vi "Date Format checkvi.vi"(1 "Date String In":string) -> (0 "Corrected Date":string)   [LabVIEW 2020]
panel:
  out "Day":string
  out "Month":string
  out "Year":string
  out "The separators are correct?":bool
  out "The year is correct?":bool
  out "The length is correct?":bool
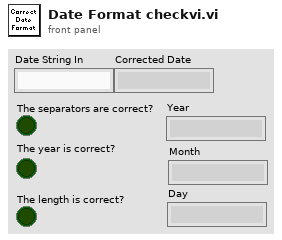
[diagram p1: front panel]
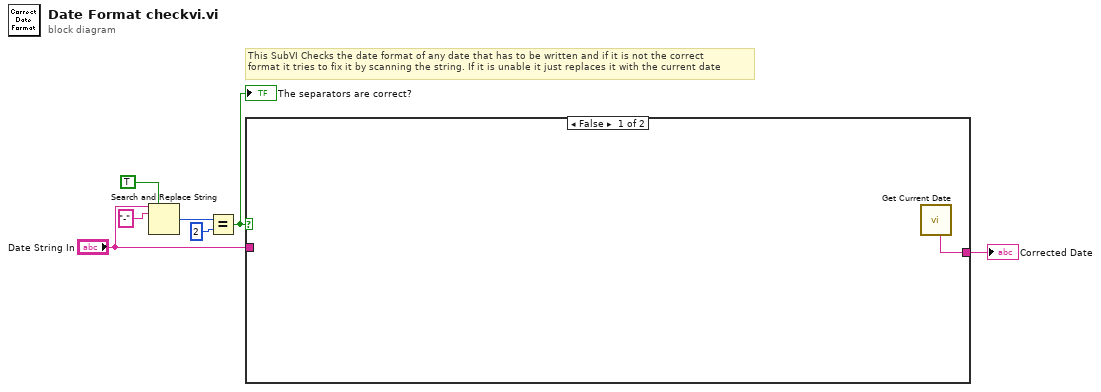
[diagram p0: block diagram]
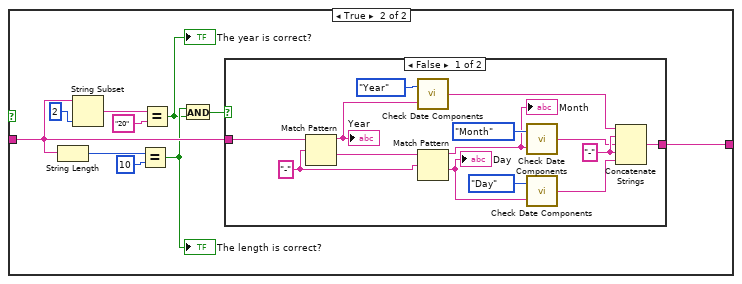
[diagram p2: hidden frame]
diagram:
  # "This SubVI Checks the date format of any date that has to be written and if it is not the correct\nformat it tries to fix it by scanning the string. If it is unable it just replaces it with the current date"
  n1 = Search and Replace String(replace all?=TRUE ("replace all? (F)"), input string="Date String In", search string="-") -> (number of replacements=w6:i32)  [unwired: 5 in, 3 out]
  n2 = Equal?(x=w6, y=2) -> (x = y?=w2:bool)
  "The separators are correct?" <- w2
  n3 = case shown="False" w2 {
    tunnel: "Date String In" -> [_ w12]
    tunnel: [w8 w13] -> w1
    frame False {
      n4 = call "Get Current Date.vi"() -> ("Formatted Current Date"=w8:string)  [unwired: 8 in, 3 out]
    }
    frame True {
      n5 = String Length(string=w12) -> (length=w17:i32)
      n6 = String Subset(string=w12, length (rest)=2 ("length (rest)")) -> (substring=w18:string)  [unwired: 1 in]
      n7 = Equal?(x=w17, y=10) -> (x = y?=w11:bool)
      "The length is correct?" <- w11
      n8 = Equal?(x=w18, y="20") -> (x = y?=w10:bool)
      "The year is correct?" <- w10
      n9 = And(x=w11, y=w10) -> (x .and. y?=w9:bool)
      n10 = case shown="False" w9 {
        tunnel: w12 -> [w32 w33]
        tunnel: [w20 w33] -> w13
        frame False {
          w19 = "-" ("search string")
          w23 = "-" ("string")
          n11 = Match Pattern(string=w32, regular expression=w19) -> (before substring=w30:string, after substring=w31:string)  [unwired: 1 in, 2 out]
          "Year" <- w30
          n12 = call "Check Date Components.vi"("Input String"=w30, "Date Type"=enum16{"Year", "Month", "Day"}."Year") -> ("Output String"=w24:string)
          n13 = Match Pattern(string=w31, regular expression=w19) -> (before substring=w25:string, after substring=w26:string)  [unwired: 1 in, 2 out]
          "Month" <- w25
          "Day" <- w26
          n14 = call "Check Date Components.vi"("Input String"=w25, "Date Type"=enum16{"Year", "Month", "Day"}."Month") -> ("Output String"=w22:string)
          n15 = call "Check Date Components.vi"("Input String"=w26, "Date Type"=enum16{"Year", "Month", "Day"}."Day") -> ("Output String"=w21:string)
          n16 = Concatenate Strings(w24, w23, w22, w23, w21) -> (w20:string)
        }
        frame True {
        }
      }
    }
  }
  "Corrected Date" <- w1
